vi "FTW-ActorConfig-FormatIdentity.vi"(0 "FTW Config String In":string="{}", 7 "Identity":string, 11 "error in":errorcluster) -> (4 "FTW Config String":string, 15 "error out":errorcluster)   [LabVIEW 2015]
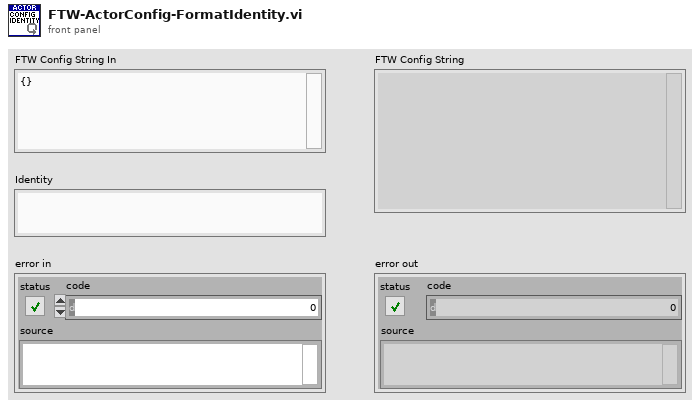
[diagram p1: front panel]
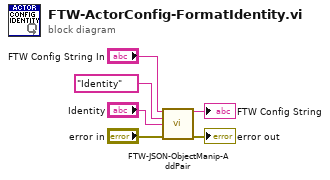
[diagram p0: block diagram]
diagram:
  n1 = call "FTW-JSON-ObjectManip-AddPair.vi"("Input JSON Object"="FTW Config String In", "Key"="Identity", "Value"="Identity", "error in"="error in") -> ("Output JSON Object"=→"FTW Config String":string, "error out"=→"error out":errorcluster)  [unwired: 10 in]
